vi "GetAxis.vi"(8 "error in (no error)":errorcluster, 10 "nodeId":u16, 11 "keyHandle in":u32) -> (0 "error out":errorcluster, 3 "axis out":cluster{"keyHandle":u32, "nodeId":u16}={"keyHandle"=0, "nodeId"=1})   [LabVIEW 2017, in "maxonEPOS.lvlib"]
doc: "<B>GetAxis</B> returns axis information."
uses:
  Examples/maxonEPOS.lvlib
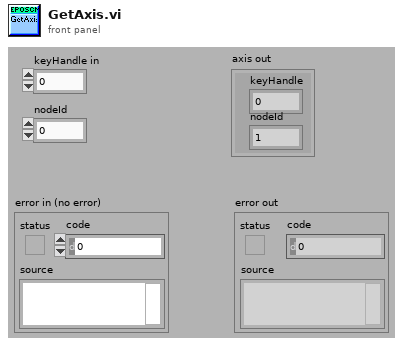
[diagram p1: front panel]
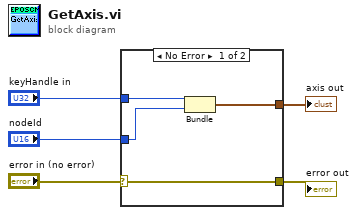
[diagram p0: block diagram]
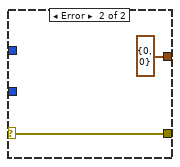
[diagram p2: hidden frame]
diagram:
  n1 = case shown="No Error" "error in (no error)" {
    selector: "error in (no error)" -> [w9 w11]
    tunnel: [w9 w11] -> w4
    tunnel: [w6 cluster{"keyHandle":u32, "nodeId":u16} {"keyHandle"=0, "nodeId"=0}] -> w1
    tunnel: "keyHandle in" -> [w8 _]
    tunnel: "nodeId" -> [w7 _]
    frame No Error {
      n2 = Bundle("keyHandle in"=w8, "nodeId"=w7) -> (w6:cluster{"keyHandle in":u32, "nodeId":u16})  [unwired: 1 in]
    }
    frame Error {
    }
  }
  "axis out" <- w1
  "error out" <- w4
